vi "File Dialog Momento.vi"(10 "Option":T1(ring) caption="Enum 3") -> (2 "Success":bool, 3 "Selected Path":path)   [LabVIEW 2024]
uses:
  <vilib>/Utility/sysdir.llb/System Directory Type.ctl
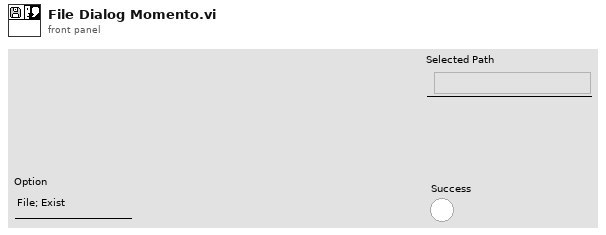
[diagram p1: front panel]
types:
  T1 = enum16{"File; Exist", "File; New or Exist", "Folder; Exist", "Folder; New or Exist"}
  T2 = typedef "System Directory Type.ctl" = i32
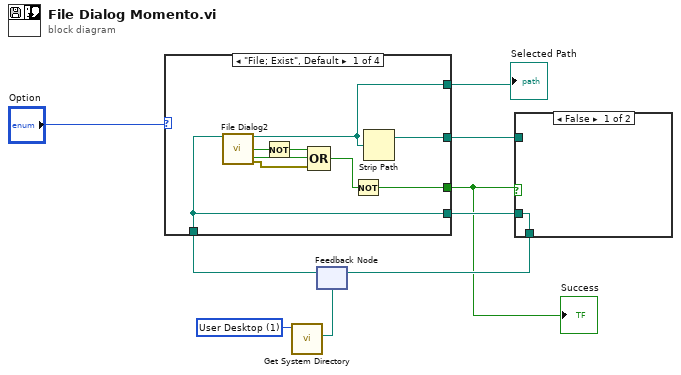
[diagram p0: block diagram]
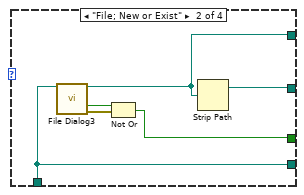
[diagram p2: hidden frame]
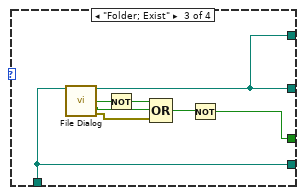
[diagram p3: hidden frame]
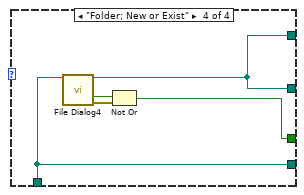
[diagram p4: hidden frame]
diagram:
  w9 = T2 1 items=["User Home"=0, "User Desktop"=1, "User Documents"=2, "User Application Data"=3, "User Preferences"=4, "User Temporary"=5, "Public Documents"=6, "Public Application Data"=7, "Public Preferences"=8, "Public Cache"=13, "System Core Libraries"=9, "System Installed Libraries"=10, "Application Files"=11, "Boot Volume Root"=12] ("system directory type")
  n1 = call <vilib>:"Get System Directory.vi"("system directory type"=w9) -> ("system directory"=w8:path)  [unwired: 10 in]
  n2 = feedback #1(w8) -> (w7:path)
  n3 = case shown="\"File; Exist\", Default" "Option" {
    tunnel: w7 -> [w16 w22 w31 w36]
    tunnel: [w18 w24 w32 w37] -> w6
    tunnel: [w17 w23 w32 w37] -> w4
    tunnel: [w16 w22 w31 w36] -> w5
    tunnel: [w10 w19 w25 w33] -> w1
    frame "File; Exist", Default {
      n4 = call "File Dialog2"("start path"=w16) -> ("selected path"=w18:path, "exists"=w15:bool, "cancelled"=w13:bool, "error out"=w12:errorcluster)  [unwired: 11 in]
      n5 = Not(x=w15) -> (.not. x?=w14:bool)
      n6 = Compound Arithmetic op=OR(w14, w13, w12) -> (w11:bool)
      n7 = Not(x=w11) -> (.not. x?=w10:bool)
      n8 = Strip Path(path=w18) -> (stripped path=w17:path)  [unwired: 1 out]
    }
    frame "File; New or Exist" {
      n9 = call "File Dialog3"("start path"=w22) -> ("selected path"=w24:path, "cancelled"=w20:bool, "error out"=w21:errorcluster)  [unwired: 11 in, 1 out]
      n10 = Not Or(1:w21, 2:w20) -> (0:w19:bool)
      n11 = Strip Path(path=w24) -> (stripped path=w23:path)  [unwired: 1 out]
    }
    frame "Folder; Exist" {
      n12 = call "File Dialog"("start path"=w31) -> ("selected path"=w32:path, "exists"=w29:bool, "cancelled"=w28:bool, "error out"=w27:errorcluster)  [unwired: 11 in]
      n13 = Not(x=w29) -> (.not. x?=w30:bool)
      n14 = Compound Arithmetic op=OR(w30, w28, w27) -> (w26:bool)
      n15 = Not(x=w26) -> (.not. x?=w25:bool)
    }
    frame "Folder; New or Exist" {
      n16 = call "File Dialog4"("start path"=w36) -> ("selected path"=w37:path, "cancelled"=w34:bool, "error out"=w35:errorcluster)  [unwired: 11 in, 1 out]
      n17 = Not Or(1:w35, 2:w34) -> (0:w33:bool)
    }
  }
  "Selected Path" <- w6
  "Success" <- w1
  n18 = case shown="False" w1 {
    tunnel: w5 -> [w38 _]
    tunnel: w4 -> [_ w39]
    tunnel: [w38 w39] -> w3
    frame False {
    }
    frame True {
    }
  }
  n19 = feedback-in #1(w3) -> ()
